vi "Get Cell Value.vi"(8 "error in":errorcluster, 9 "Cell Address":string, 10 "Sheet Name":string, 11 "SpreadsheetDocument":refnum<k24>) -> (0 "error out":errorcluster, 1 "Value Numeric":dbl, 2 "Value String":string, 3 "SpreadsheetDocument out":refnum<k24>, 4 "Type":enum16{"String", "Numeric"}(ring))   [LabVIEW 2021, in "Open Xml.lvlib"]
uses:
  Open Xml.lvlib
  D:/git/Open-Xml-LabVIEW/DocumentFormat.OpenXml.dll
  DocumentFormat.OpenXml.dll
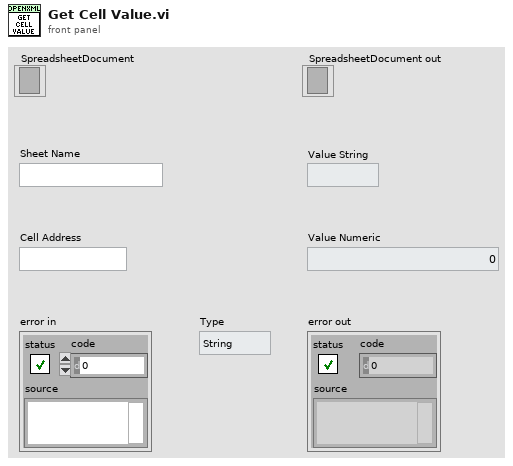
[diagram p1: front panel]
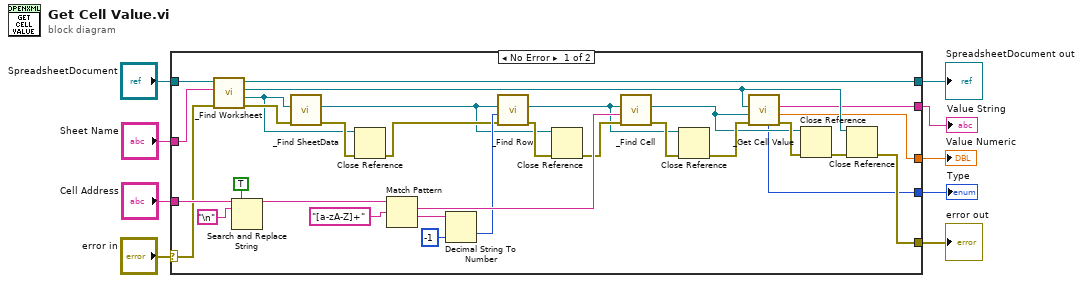
[diagram p0: block diagram]
diagram:
  n1 = case shown="No Error" "error in" {
    selector: "error in" -> [w31 w42]
    tunnel: "Sheet Name" -> [w40 _]
    tunnel: "Cell Address" -> [w38 _]
    tunnel: [w20 w42] -> w6
    tunnel: "SpreadsheetDocument" -> [w18 w41]
    tunnel: [w16 w41] -> w4
    tunnel: [w15 _] -> w2
    tunnel: [w14 _] -> w3
    tunnel: [w13 _] -> w1
    frame No Error {
      n2 = call "_Find Worksheet.vi"("error in"=w31, "Sheet Name"=w40, "SpreadsheetDocument"=w18) -> ("error out"=w39:errorcluster, "Worksheet"=w26:refnum<k24>, "WorkbookPart"=w17:refnum<k24>, "SpreadsheetDocument out"=w16:refnum<k24>)  [unwired: 5 in]
      n3 = Search and Replace String(replace all?=TRUE ("replace all? (F)"), input string=w38, search string="\n") -> (result string=w12:string)  [unwired: 5 in, 3 out]
      n4 = call "_Find SheetData.vi"("error in"=w39, "Worksheet"=w26) -> ("error out"=w30:errorcluster, "SheetData"=w24:refnum<k24>)  [unwired: 8 in]
      n5 = Close Reference(reference=w26, error in (no error)=w30) -> (error out=w27:errorcluster)
      n6 = Match Pattern(string=w12, regular expression="[a-zA-Z]+") -> (match substring=w36:string, after substring=w35:string)  [unwired: 1 in, 2 out]
      n7 = Decimal String To Number(string=w35, default (0L)=-1 ("default (0 I32)")) -> (number=w34:i32)  [unwired: 1 in, 1 out]
      n8 = call "_Find Row.vi"("error in"=w27, "Index"=w34, "SheetData"=w24) -> ("error out"=w28:errorcluster, "Row"=w22:refnum<k24>)  [unwired: 7 in]
      n9 = Close Reference(reference=w24, error in (no error)=w28) -> (error out=w25:errorcluster)
      n10 = call "_Find Cell.vi"("error in"=w25, "Lexical Index"=w36, "Row"=w22) -> ("error out"=w29:errorcluster, "Cell"=w19:refnum<k24>)  [unwired: 7 in]
      n11 = Close Reference(reference=w22, error in (no error)=w29) -> (error out=w23:errorcluster)
      n12 = call "_Get Cell Value.vi"("error in"=w23, "Cell"=w19, "Workbookpart"=w17) -> ("error out"=w32:errorcluster, "Value Numeric"=w15:dbl, "Value String"=w13:string, "Type"=w14:enum16{"String", "Numeric"})  [unwired: 5 in]
      n13 = Close Reference(reference=w19, error in (no error)=w32) -> (error out=w21:errorcluster)
      n14 = Close Reference(reference=w17, error in (no error)=w21) -> (error out=w20:errorcluster)
    }
    frame Error {
    }
  }
  "error out" <- w6
  "SpreadsheetDocument out" <- w4
  "Type" <- w3
  "Value Numeric" <- w2
  "Value String" <- w1
